vi "Configure Protection.vi"(6 "Protection (None)":T1, 8 "error in":errorcluster, 10 "Limit":dbl, 11 "9115AT in":refnum<class "9115AT.lvclass">) -> (0 "error out":errorcluster, 3 "9115AT out":refnum<class "9115AT.lvclass">)   [LabVIEW 2018, in "9115AT.lvlib" / "9115AT.lvclass"]
doc: "Configure Protection setting, available options:\n\n0: None\n1: Over Voltage\n2: Under Voltage\n3: Over Current\n\nDbl Precision Limit"
uses:
  9115AT.lvclass
  builds/Power_Supply.lvlibp/Custom Control/Protection.ctl
  <instrlib>/BK Precision 911X Series/BK Precision 911X Series.lvlib
  builds/Power_Supply.lvlibp/Power Supply.lvclass
  C:/Users/Ron.Dexter.LUMINARTECH/Desktop/builds/Power_Supply.lvlibp/Power Supply.lvclass
  builds/Power_Supply.lvlibp
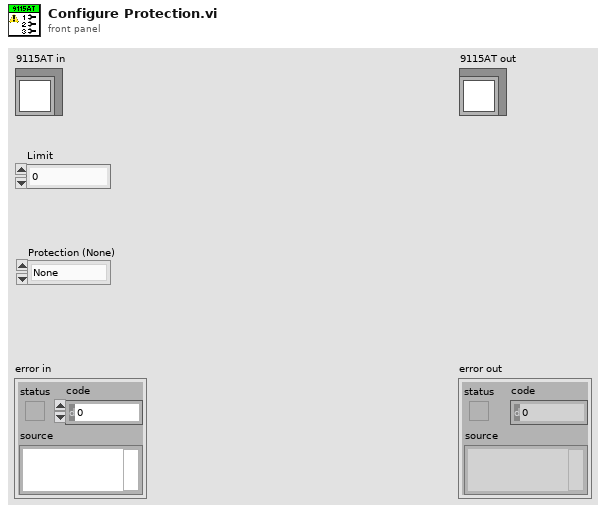
[diagram p1: front panel]
types:
  T1 = typedef "Power_Supply.lvlibp/Protection.ctl" = enum16{"None", "Over Volt", "Under Volt", "Over Current"}
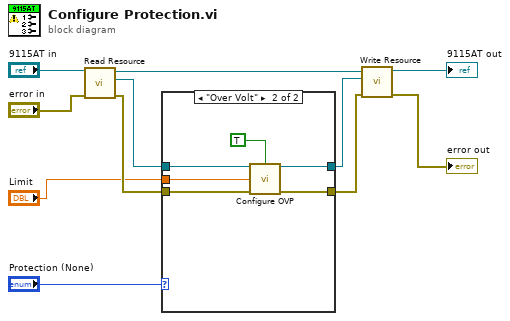
[diagram p0: block diagram]
diagram:
  n1 = call "Read Resource.vi"("error in"="error in", "Power Supply in"="9115AT in") -> ("error out"=w5:errorcluster, "Resource"=w7:refnum<visa-resource-name>, "Power Supply out"=w10:refnum<class "9115AT.lvclass">)  [unwired: 7 in]
  n2 = case shown="\"Over Volt\"" "Protection (None)" {
    tunnel: w7 -> [w13 w19]
    tunnel: [w13 w18] -> w6
    tunnel: w5 -> [w12 w17]
    tunnel: [w12 w16] -> w4
    tunnel: "Limit" -> [_ w15]
    frame "None", Default {
    }
    frame "Over Volt" {
      n3 = call <instrlib>:"Configure OVP.vi"("VISA resource name"=w19, "Enable OVP (T: Enable)"=TRUE, "Voltage Limit (80.000 V)"=w15, "error in (no error)"=w17) -> ("VISA resource name out"=w18:refnum<visa-resource-name>, "error out"=w16:errorcluster)  [unwired: 10 in]
    }
  }
  n4 = call "Write Resource.vi"("error in"=w4, "Resource"=w6, "Power Supply in"=w10) -> ("error out"=→"error out":errorcluster, "Power Supply out"=→"9115AT out":refnum<class "9115AT.lvclass">)  [unwired: 7 in]
